vi "Main.vi"() -> ()   [LabVIEW 2025, in "Status Log.lvlib"]
uses:
  Status Log.lvlib
panel:
  out "Status Messages":string
  out "Status Log Path":path
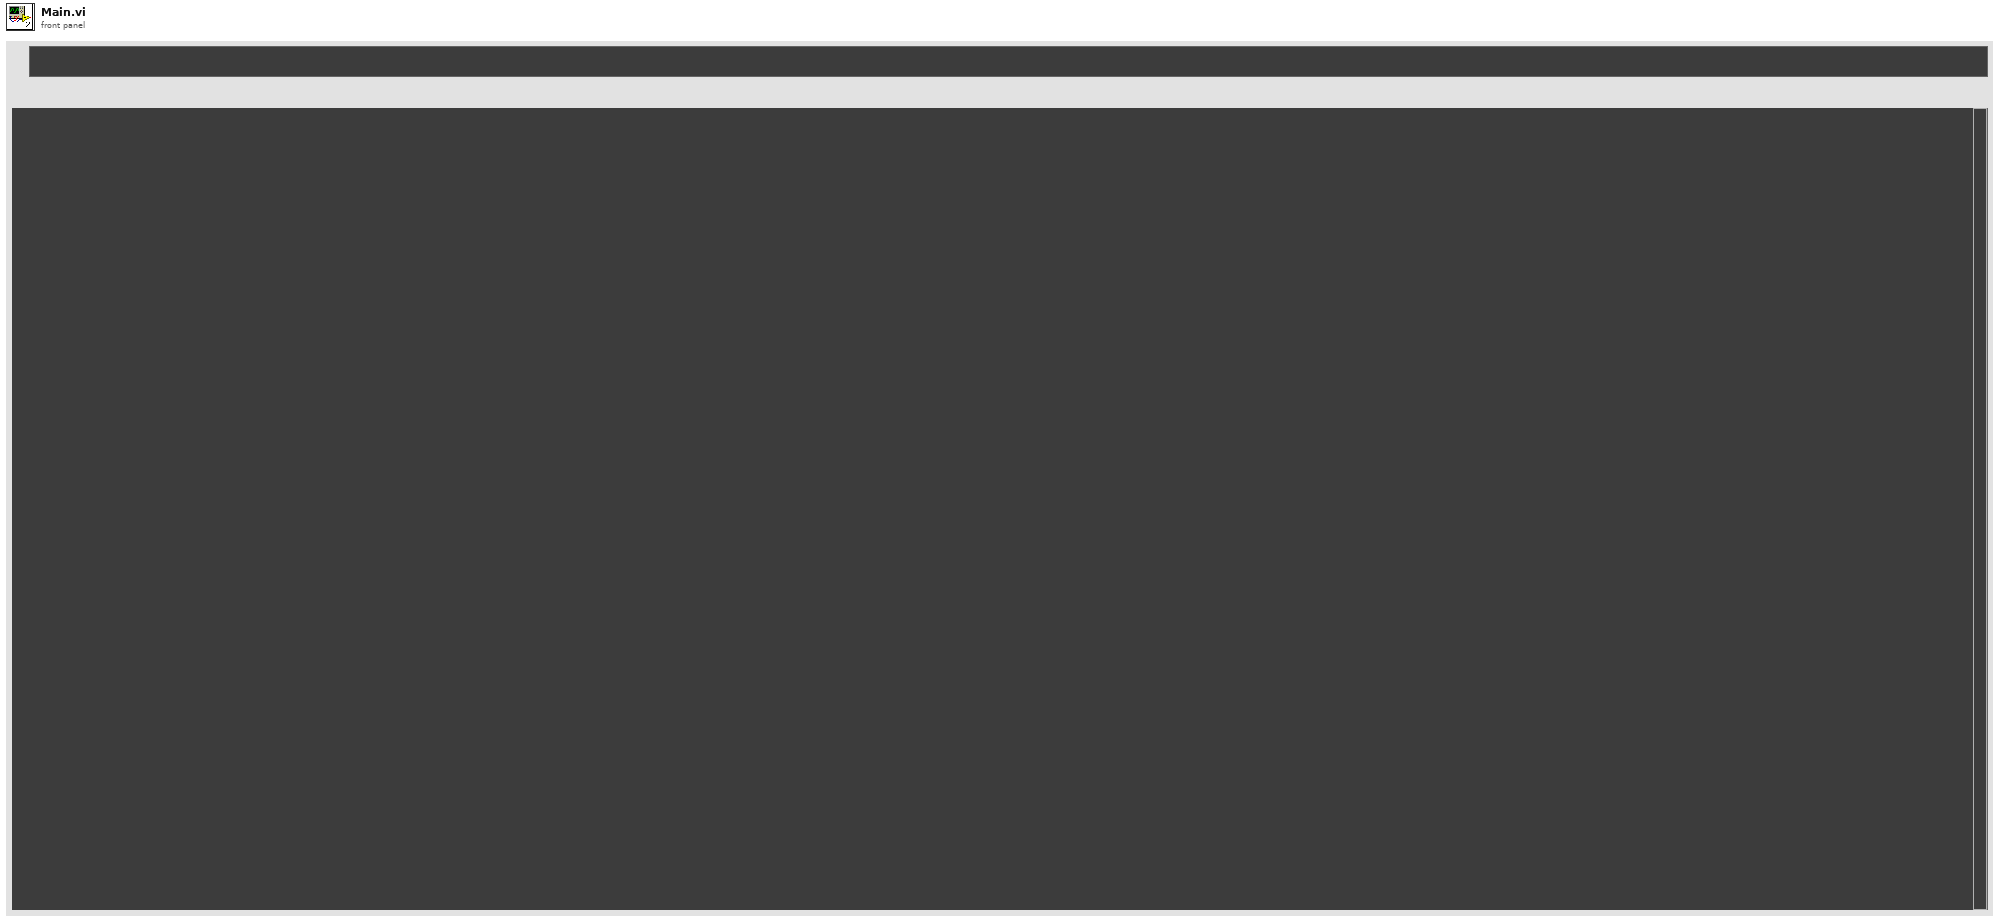
[diagram p1: front panel]
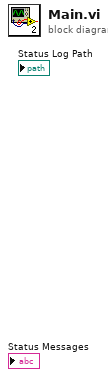
[diagram p0: block diagram]
diagram:
